vi "circ_ap && forvard.vi"() -> ()   [LabVIEW 2012, in "LightPipes.lvlib"]
uses:
  LightPipes.lvlib
panel:
  in  "distance":dbl=1.0
  out "Field":cluster{"n_grid":i32, "size":dbl, "lambda":dbl}
  # "Forward"
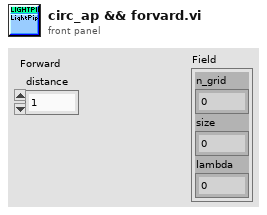
[diagram p1: front panel]
types:
  T1 = cluster{"n_grid":i32, "@dummy control@":i8, "@dummy control@":i8, "@dummy control@":i8, "@dummy control@":i8, "size":dbl, "lambda":dbl, "int1":i32, "int2":i32, "int3":i32, "@dummy control@":i8, "@dummy control@":i8, "@dummy control@":i8, "@dummy control@":i8, "double1":dbl, "double2":dbl, "double3":dbl, "real":u32, "imaginary":u32}
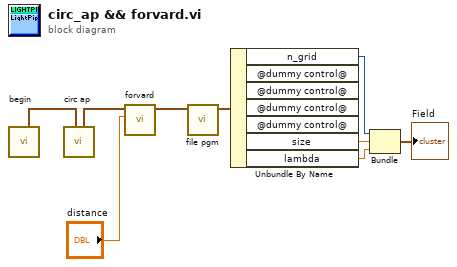
[diagram p0: block diagram]
diagram:
  n1 = call "begin.vi"() -> ("field out"=w5:T1)  [unwired: 11 in]
  n2 = call "circ ap.vi"("field"=w5) -> ("field out"=w4:T1)  [unwired: 10 in]
  n3 = call "forvard.vi"("distance"="distance", "field"=w4) -> ("field out"=w2:T1)  [unwired: 9 in]
  n4 = call "file pgm.vi"("field"=w2) -> ("field out"=w1:T1)  [unwired: 9 in, 1 out]
  n5 = Unbundle By Name(w1) -> ("n_grid"=w6:i32, "size"=w7:dbl, "lambda"=w8:dbl)  [unwired: 4 out]
  n6 = Bundle("n_grid"=w6, "size"=w7, "lambda"=w8) -> (→"Field":cluster{"n_grid":i32, "size":dbl, "lambda":dbl})  [unwired: 1 in]
